vi "Queue test.vi"() -> ()   [LabVIEW 2017]
panel:
  out "Array":dbl[][](array[numeric])
  out "# elements in queue":i32
  out "TempData":bool=TRUE
  in  "temp typedef":dbl[][](array[numeric])
  in  "Array 5":dbl[][](array[numeric])
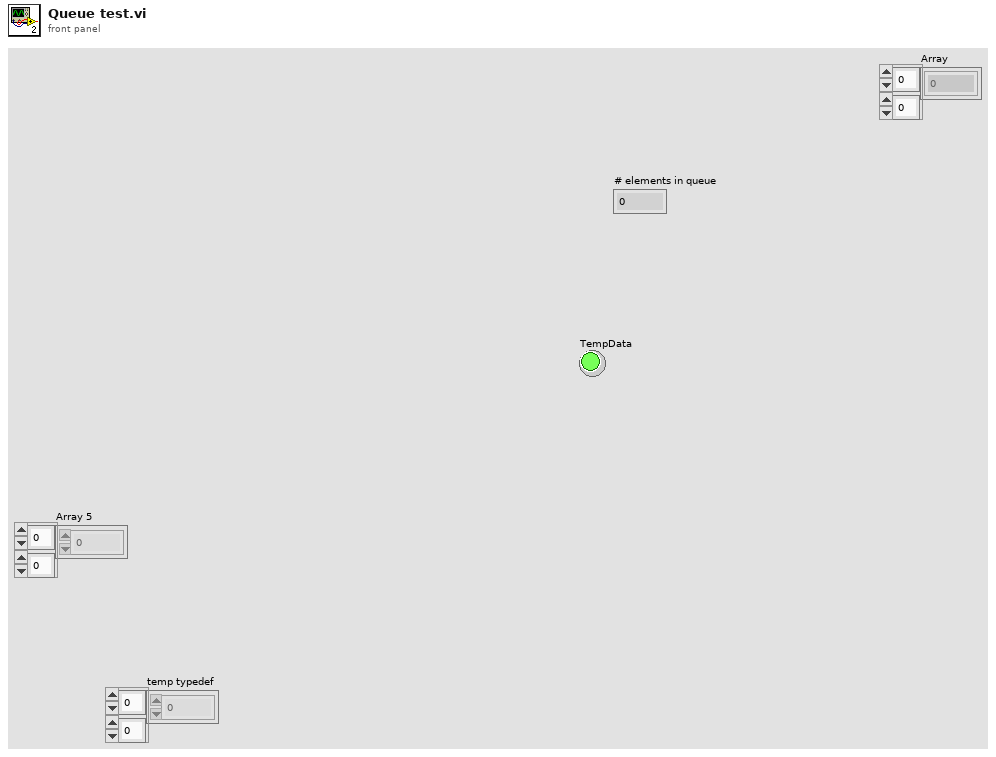
[diagram p1: front panel]
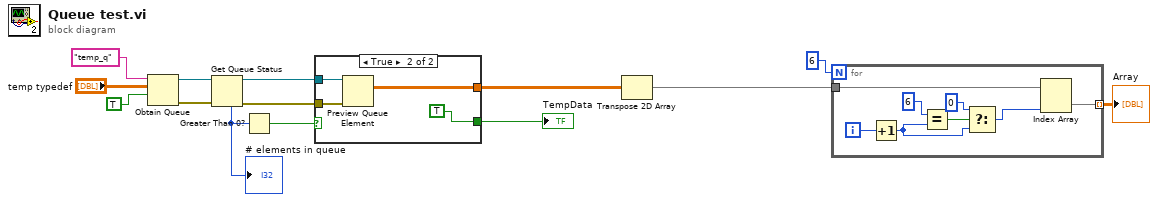
[diagram p0: block diagram]
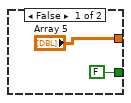
[diagram p2: hidden frame]
diagram:
  n1 = Obtain Queue(name (unnamed)="temp_q", element data type="temp typedef", create if not found? (T)=TRUE) -> (queue out=w6:refnum<queue>, error out=w7:errorcluster)  [unwired: 2 in, 1 out]
  n2 = Get Queue Status(queue=w6, error in (no error)=w7) -> (queue out=w12:refnum<queue>, error out=w13:errorcluster, # elements in queue=w14:i32)  [unwired: 1 in, 5 out]
  "# elements in queue" <- w14
  n3 = Greater Than 0?(x=w14) -> (x > 0?=w11:bool)
  n4 = case shown="True" w11 {
    tunnel: w13 -> [_ w19]
    tunnel: w12 -> [_ w20]
    tunnel: ["Array 5" w18] -> w4
    tunnel: [FALSE TRUE] -> w5
    frame False {
    }
    frame True {
      n5 = Preview Queue Element(queue=w20, error in (no error)=w19) -> (element=w18:dbl[][])  [unwired: 1 in, 3 out]
    }
  }
  "TempData" <- w5
  n6 = Transpose 2D Array(2D array=w4) -> (transposed array=w3:dbl[][])
  n7 = for {
    N: 6 -> [_]
    tunnel: w3 -> [w27]
    tunnel: [w26] -> w1 mode=indexing
    i -> [w28]
    n8 = Increment(x=w28) -> (x+1=w21:i32)
    n9 = Equal?(x=6 ("y"), y=w21) -> (x = y?=w25:bool)
    n10 = Select(t=0, s=w25, f=w21) -> (s? t:f=w22:i32)
    n11 = Index Array(array=w27, index (col)=w22) -> (element=w26:dbl[])  [unwired: 1 in]
  }
  "Array" <- w1
